vi "OffsetArrayForStrummingPattern.vi"(10 "input array":dbl[](array[numeric]), 11 "offset":i32) -> (3 "Array":dbl[](array[numeric]))   [LabVIEW 2016]
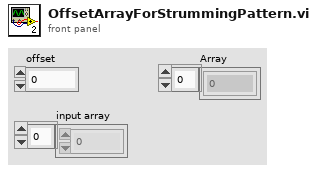
[diagram p1: front panel]
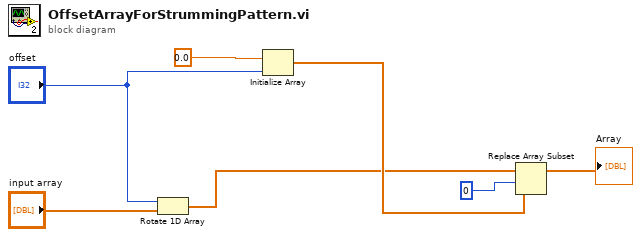
[diagram p0: block diagram]
diagram:
  n1 = Rotate 1D Array(1:"input array", 2:"offset") -> (0:w2:dbl[])
  n2 = Initialize Array(0.0 ("element"), "offset") -> (w5:dbl[])
  n3 = Replace Array Subset(array=w2, new element=w5, index=0) -> (→"Array":dbl[])
